vi "FABR-Update Stimulus.vi"(0 "Runtime in":T2, 7 "SCL in":cluster{T1[]}[](array[cluster]), 11 "error in (no error)":errorcluster, 12 "start":bool) -> (4 "Runtime out":T2, 8 "SCL out":cluster{T1[]}[](array[cluster]), 15 "error out":errorcluster)   [LabVIEW 2020]
uses:
  Typedefs/FABR-Runtime Data.ctl
  Typedefs/FABR-Stimulus Ticket.ctl
  Typedefs/FABR-Order.ctl
  Typedefs/FABR-Stimulus Condition.ctl
  epl-vi-lib/PXI DAQ VIs/AODO/Typedefs/AODO-Action.ctl
  32b95af9-b274-447d-9881-c5549455fd14.vi
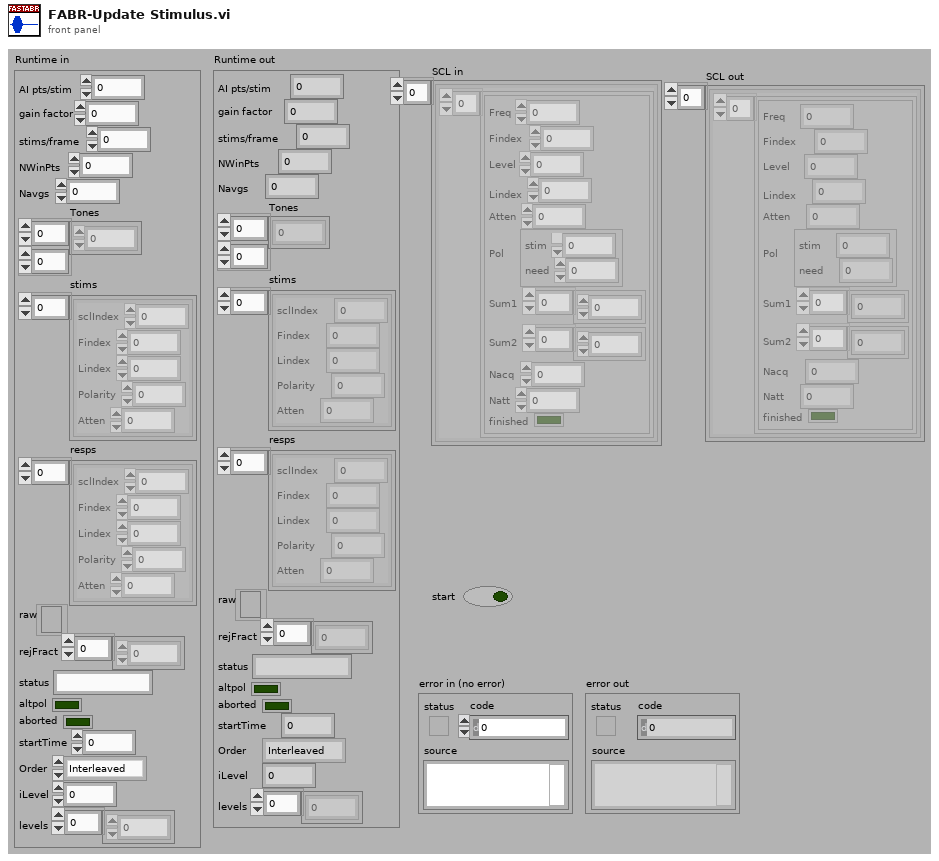
[diagram p1: front panel]
types:
  T1 = typedef "FABR-Stimulus Condition.ctl" = cluster{"Freq":dbl, "Findex":i32, "Level":dbl, "Lindex":i32, "Atten":dbl, "Pol":cluster{"stim":i32, "need":i32}, "Sum1":dbl[], "Sum2":dbl[], "Nacq":i32, "Natt":i32, "finished":bool}
  T2 = typedef "FABR-Runtime Data.ctl" = cluster{"AI pts/stim":i32, "gain factor":dbl, "stims/frame":i32, "NWinPts":i32, "Navgs":i32, "Tones":dbl[][], "stims":T3[], "resps":T3[], "raw":refnum<file>, "rejFract":dbl[], "status":string, "altpol":bool, "aborted":bool, "startTime":dbl, "Order":T4, "iLevel":i32, "levels":dbl[]}
  T3 = typedef "FABR-Stimulus Ticket.ctl" = cluster{"sclIndex":i32, "Findex":i32, "Lindex":i32, "Polarity":i32, "Atten":dbl}
  T4 = typedef "FABR-Order.ctl" = enum16{"Interleaved", "Stepped level"}
  T5 = typedef "AODO-Action.ctl" = enum16{"Configure", "Initialize", "Start", "Write", "Clean up", "Init & Start", "Config & Test", "Position", "Set AO Gains", "Zero", "Prime", "Status"}
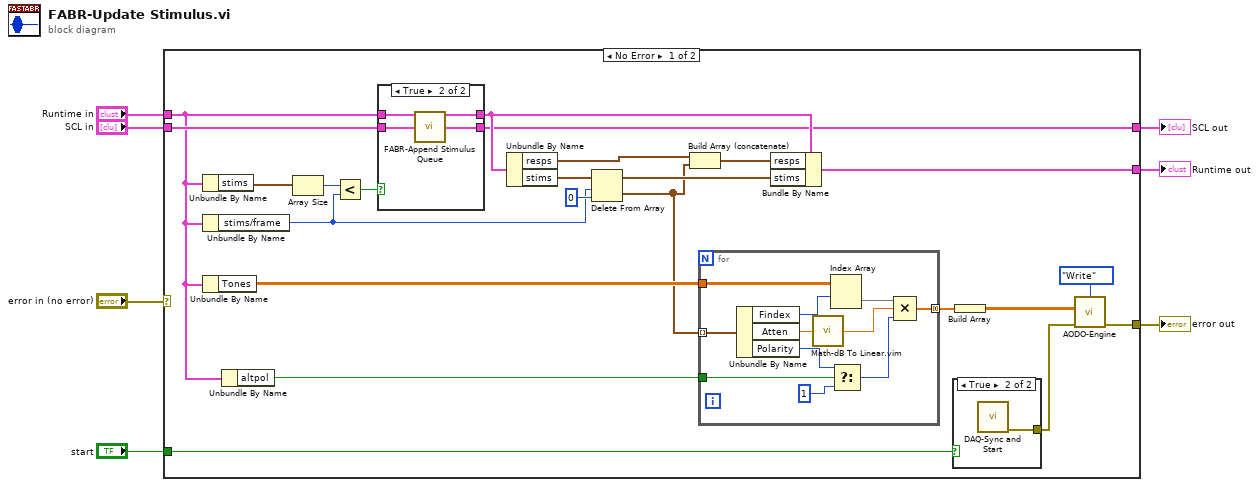
[diagram p0: block diagram]
diagram:
  n1 = case shown="No Error" "error in (no error)" {
    selector: "error in (no error)" -> [_ w51]
    tunnel: [w11 w51] -> w7
    tunnel: "Runtime in" -> [w9 w50]
    tunnel: [w17 w50] -> w4
    tunnel: "start" -> [w13 _]
    tunnel: "SCL in" -> [w27 w49]
    tunnel: [w10 w49] -> w1
    frame No Error {
      n2 = Unbundle By Name(w9) -> ("stims"=w30:T3[])
      n3 = Unbundle By Name(w9) -> ("stims/frame"=w24:i32)
      n4 = Unbundle By Name(w9) -> ("Tones"=w21:dbl[][])
      n5 = Unbundle By Name(w9) -> ("altpol"=w8:bool)
      n6 = Array Size(array=w30) -> (size(s)=w29:i32)
      n7 = Less?(x=w29, y=w24) -> (x < y?=w28:bool)
      n8 = case shown="True" w28 {
        tunnel: w9 -> [w33 w37]
        tunnel: [w33 w36] -> w23
        tunnel: w27 -> [w32 w35]
        tunnel: [w32 w34] -> w10
        frame False {
        }
        frame True {
          n9 = call "FABR-Append Stimulus Queue.vi"("Runtime in"=w37, "SCL in"=w35) -> ("Runtime out"=w36:T2, "SCL out"=w34:cluster{T1[]}[])  [unwired: 11 in, 1 out]
        }
      }
      n10 = Unbundle By Name(w23) -> ("resps"=w20:T3[], "stims"=w26:T3[])
      n11 = Delete From Array(array=w26, length=w24, index=0) -> (deleted portion=w19:T3[], array with subset deleted=w22:T3[])
      n12 = Build Array (concatenate)(w20, w19) -> (w18:T3[])
      n13 = for {
        tunnel: w19 -> [w48] mode=indexing
        tunnel: w21 -> [w47]
        tunnel: [w44] -> w16 mode=concatenating
        tunnel: w8 -> [w41]
        n14 = Unbundle By Name(w48) -> ("Findex"=w46:i32, "Atten"=w43:dbl, "Polarity"=w42:i32)
        n15 = call "Math-dB To Linear.vim"("dB"=w43) -> ("linear"=w40:dbl)
        n16 = Index Array(array=w47, index (row)=w46) -> (element=w45:dbl[])  [unwired: 1 in]
        n17 = Select(t=w42, s=w41, f=1) -> (s? t:f=w39:i32)
        n18 = Compound Arithmetic op=MULTIPLY(w45, w40, w39) -> (w44:dbl[])
      }
      n19 = Bundle By Name(cluster=w23, "resps"=w18, "stims"=w22) -> (w17:T2)
      n20 = case shown="True" w13 {
        tunnel: [_ w31] -> w12
        frame False {
        }
        frame True {
          n21 = call "DAQ-Sync and Start.vi"() -> ("error out"=w31:errorcluster)  [unwired: 15 in]
        }
      }
      n22 = Build Array(w16) -> (w15:dbl[][])
      n23 = call "AODO-Engine.vi"("Action"=AODO-Action."Write", "AO"=w15, "error in (no error)"=w12) -> ("error out"=w11:errorcluster)  [unwired: 7 in, 5 out]
    }
    frame Error {
    }
  }
  "error out" <- w7
  "Runtime out" <- w4
  "SCL out" <- w1
